vi "checkifErrorAndDisconnectsubVI.vi"() -> ()   [LabVIEW 2012]
uses:
  <userlib>/SPECcon/SPECcon.lvlib
panel:
  in  "function return":i32
  in  "port_number in":string
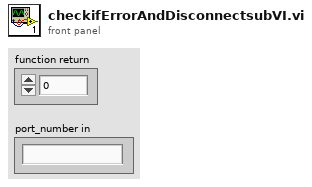
[diagram p1: front panel]
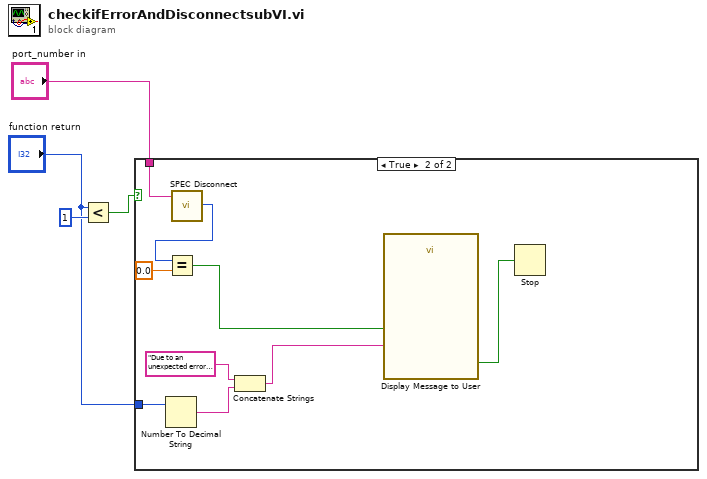
[diagram p0: block diagram]
diagram:
  n1 = Less?(x="function return", y=1) -> (x < y?=w2:bool)
  n2 = case shown="True" w2 {
    tunnel: "port_number in" -> [_ w10]
    tunnel: "function return" -> [_ w8]
    frame False {
    }
    frame True {
      n3 = Number To Decimal String(number=w8) -> (decimal integer string=w7:string)  [unwired: 1 in]
      n4 = call <userlib>:"SPEC Disconnect.vi"("port_number"=w10) -> ("function return"=w9:i32)  [unwired: 9 in, 1 out]
      n5 = Equal?(x=w9, y=0.0) -> (x = y?=w13:bool)
      n6 = Concatenate Strings("Due to an unexpected error, spectrometer is disconnected. Please rerun the program and reconnect.\n\nError Code: ", w7) -> (w6:string)
      n7 = call "Display Message to User"("Enable"=w13, "Message"=w6) -> ("OK"=w11:bool)  [unwired: 8 in, 1 out]
      n8 = Stop(stop? (T)=w11) -> ()
    }
  }
